vi "AMC Queue Registry.vi"(6 "Properties in":T1, 8 "error in (no error)":errorcluster, 9 "Message Queue in":T2, 10 "Index":i32, 11 "Method":T3) -> (0 "error out":errorcluster, 1 "Message Queue out":T2, 2 "Number of Queues":i32, 3 "All Queues":T2[](array[typedef]), 4 "Properties out":T1, 5 "All Properties":T1[](array[typedef]))   [LabVIEW 2015]
doc: "This VI is used for compatibility with previous versions of the AMC library. Use the AMC VIs located in the <b>Data Communication >> Asynchronous Message Communication</b> palette."
uses:
  <vilib>/NI/AMC/Queue Registry Method.ctl
  <vilib>/NI/AMC/Message Queue.ctl
  <vilib>/NI/AMC/Message.ctl
  <vilib>/NI/Tools/Keyed Array/KeyedArray.ctl
  <vilib>/NI/AMC/Queue Registry Properties.ctl
  <vilib>/NI/AMC/AMC.lvlib
  <vilib>/NI/Tools/Keyed Array/Tools_KeyedArray.lvlib
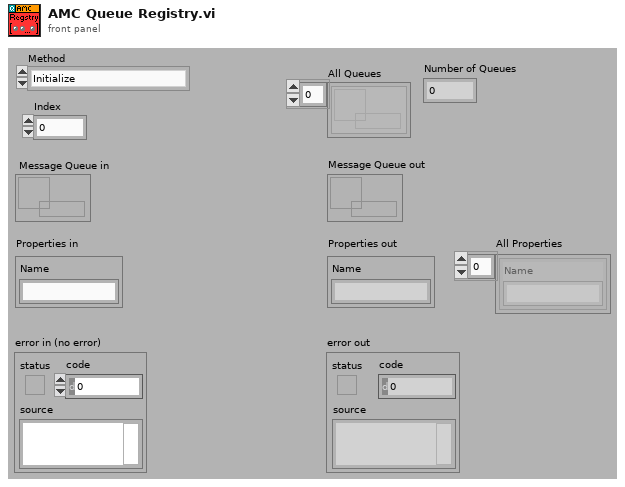
[diagram p1: front panel]
types:
  T1 = typedef "AMC.lvlib/Queue Registry Properties.ctl" = cluster{"Name":string}
  T2 = typedef "AMC.lvlib/Message Queue.ctl" = refnum<queue>
  T3 = typedef "AMC.lvlib/Queue Registry Method.ctl" = enum16{"Initialize", "Add Queue", "Set Properties", "Get Queue by Index", "Get Queue by Name", "Remove Queue", "Remove All Queues"}
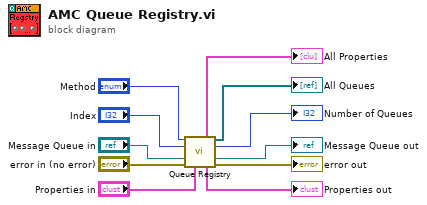
[diagram p0: block diagram]
diagram:
  n1 = call <vilib>:"Queue Registry.vi"("method"="Method", "index (0)"="Index", "message queue in"="Message Queue in", "error in"="error in (no error)", "properties in"="Properties in") -> ("all properties"=→"All Properties":T1[], "all queues"=→"All Queues":T2[], "number of queues"=→"Number of Queues":i32, "message queue out"=→"Message Queue out":T2, "properties out"=→"Properties out":T1, "error out"=→"error out":errorcluster)  [unwired: 5 in]
